vi "Check for Digital Trigger.vi"(8 "error in (no error)":errorcluster, 11 "4300 in":refnum<class "4300.lvclass">) -> (0 "error out":errorcluster, 1 "TriggerSource":string, 2 "IsDigital":bool, 3 "4300 out":refnum<class "4300.lvclass">)   [LabVIEW 2019, in "4300.lvlib" / "4300.lvclass"]
uses:
  Library/4300.lvclass
  C:/Users/Public/Documents/Development/builds/Instruments/AnalogInput.lvlibp/Library/AnalogInput.lvclass
  builds/Instruments/AnalogInput.lvlibp/Accessors/Triggering/Read DIG_TRIG_SRC.vi
  builds/Instruments/AnalogInput.lvlibp/Accessors/Triggering/Read DIG_TRIG_NAME.vi
  builds/Instruments/AnalogInput.lvlibp/Accessors/Triggering/Read Trigger Source.vi
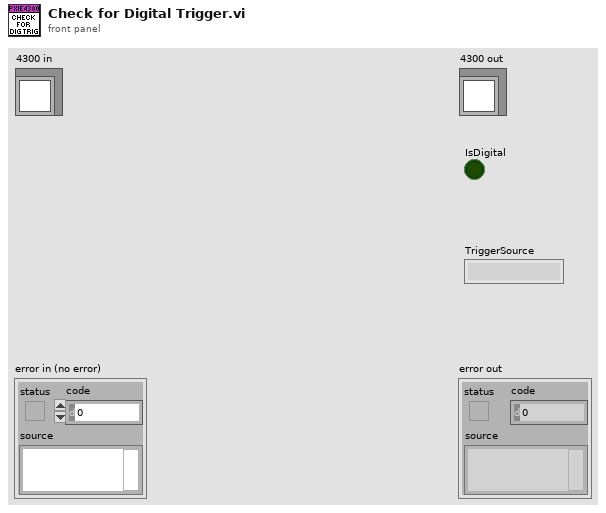
[diagram p1: front panel]
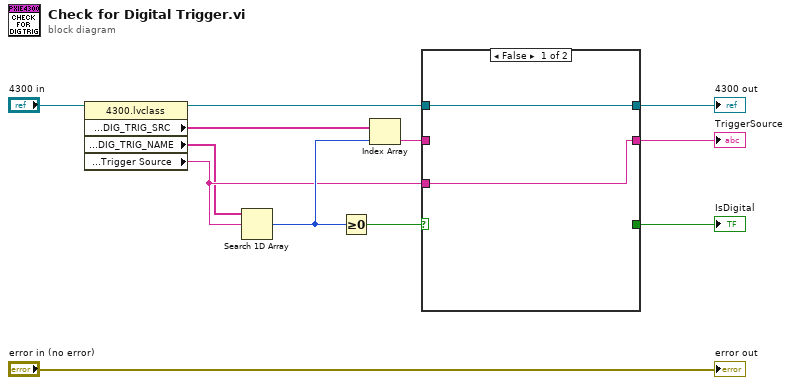
[diagram p0: block diagram]
diagram:
  n1 = property class="4300.lvclass"(reference="4300 in") -> (reference out=w10:refnum<class "4300.lvclass">, "Accessors:Triggering:DIG_TRIG_SRC"=w1:string[], "Accessors:Triggering:DIG_TRIG_NAME"=w2:string[], "Accessors:Triggering:Trigger Source"=w5:string)  [unwired: 1 in, 1 out]
  n2 = Search 1D Array(1D array=w2, element=w5) -> (index of element=w9:i32)  [unwired: 1 in]
  n3 = Greater Or Equal To 0?(x=w9) -> (x >= 0?=w8:bool)
  n4 = Index Array(array=w1, index=w9) -> (element=w7:string)
  n5 = case shown="False" w8 {
    selector: w8 -> [_ w15]
    tunnel: w10 -> [w13 w17]
    tunnel: w7 -> [_ w16]
    tunnel: [w13 w17] -> w6
    tunnel: [w14 w16] -> w3
    tunnel: w5 -> [w14 _]
    tunnel: [_ w15] -> w4
    frame False {
    }
    frame True {
    }
  }
  "4300 out" <- w6
  "IsDigital" <- w4
  "TriggerSource" <- w3
  "error out" <- "error in (no error)"
